vi "Broadcast SensorInfo.vi"(8 "error in (no error)":errorcluster, 11 "Sensor in":refnum<class "Sensor.lvclass">) -> (0 "error out":errorcluster, 3 "Sensor out":refnum<class "Sensor.lvclass">)   [LabVIEW 2012, in "Sensor Definition.lvlib" / "Sensor.lvclass"]
uses:
  Sensor.lvclass
  Sensor.lvclass/Sensor.ctl
  SensorView Messages/Update Sensor Info Msg/Update Sensor Info Msg.lvclass/Update Sensor Info Msg.ctl
  <vilib>/ActorFramework/Message Enqueuer/Message Enqueuer.lvclass/Message Enqueuer.ctl
  Read Listening SensorViews.vi
  Read SensorInfo.vi
  <vilib>/ActorFramework/Message Enqueuer/Enqueue.vi
  <vilib>/ActorFramework/Message Priority Queue/Priority Enqueue.vi
  <vilib>/ActorFramework/Message Enqueuer/Message Enqueuer.lvclass
  SensorInfo.lvclass
  SensorView Messages/Update Sensor Info Msg/Update Sensor Info Msg.lvclass
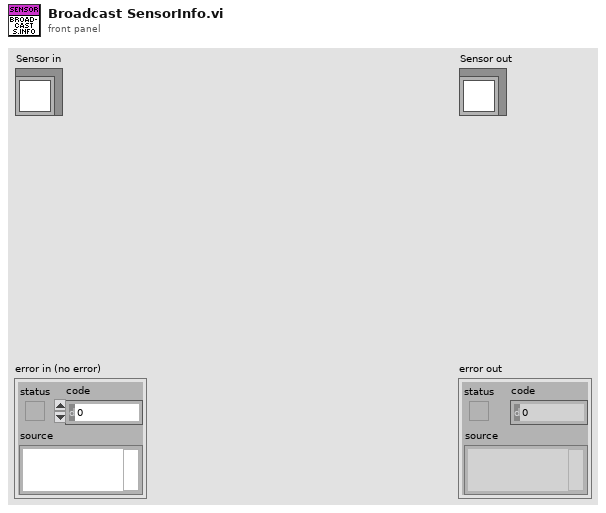
[diagram p1: front panel]
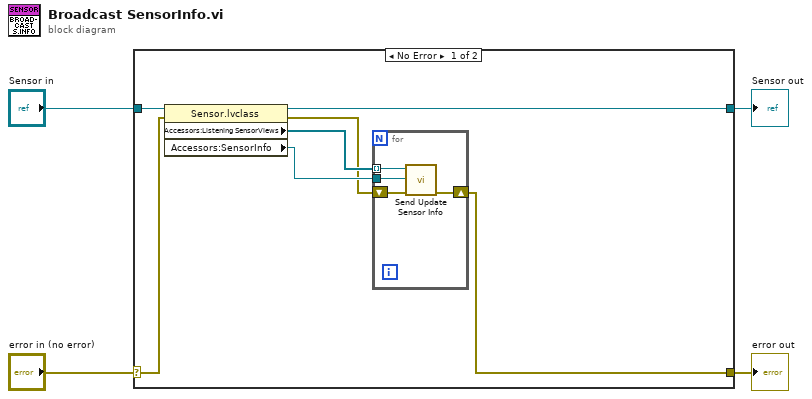
[diagram p0: block diagram]
diagram:
  n1 = case shown="No Error" "error in (no error)" {
    selector: "error in (no error)" -> [w6 w17]
    tunnel: [w7 w17] -> w3
    tunnel: [w10 w16] -> w1
    tunnel: "Sensor in" -> [w11 w16]
    frame No Error {
      n2 = property class="Sensor.lvclass"(reference=w11, error in=w6) -> (reference out=w10:refnum<class "Sensor.lvclass">, error out=w5:errorcluster, "Accessors:Listening SensorViews"=w9:refnum<class "Message Enqueuer.lvclass">[], "Accessors:SensorInfo"=w8:refnum<class "SensorInfo.lvclass">)
      n3 = for {
        tunnel: w9 -> [w15] mode=indexing
        tunnel: w8 -> [w14]
        shift-right: [w12] -> w7
        shift-left: w5 -> [w13]
        n4 = call "Send Update Sensor Info.vi"("error in (no error)"=w13, "SensorInfo"=w14, "Message Enqueuer"=w15) -> ("error out"=w12:errorcluster)  [unwired: 7 in, 1 out]
      }
    }
    frame Error {
    }
  }
  "error out" <- w3
  "Sensor out" <- w1
